vi "3D Omni Robot.vi"() -> ()   [LabVIEW 2015]
doc: "This example shows how to use the Steering VIs to define and simulate a dynamic model of a three-wheeled omnidirectional robot on a smooth surface."
uses:
  Robot Position.ctl
  <vilib>/robotics/Steering/Wheel/Wheel Parameters.ctl
  <vilib>/robotics/Steering/Wheel/Rotation Direction.ctl
  <vilib>/Simulation/Scripting/Companion Diagram/SimConfigNode/SimParams.ctl
  <vilib>/Simulation/Scripting/Companion Diagram/SimConfigNode/_simSolvers.ctl
  <vilib>/Simulation/Implementation/Shared/SIMSCR Execution Mode.ctl
  <vilib>/Platform/TimedLoop/XDataNode/timing_clust.ctl
  <vilib>/Platform/TimedLoop/XDataNode/nitl_modes.ctl
  <vilib>/Platform/TimedLoop/XDataNode/wakeup.ctl
  <vilib>/Simulation/Param Hierarchy/Typedefs/SIMPH Param Control Actions.ctl
  <vilib>/Simulation/Implementation/Shared/NILVSim_ParamChanged.vi
  <vilib>/Simulation/Implementation/Shared/NILVSim_FinishedLate.vi
  <vilib>/Simulation/Implementation/Shared/NILVSIM_BeginStep.vi
  <vilib>/Simulation/Utility/Implementation/SIM Halt.vi
  <vilib>/Simulation/Implementation/Shared/NILVSim_Manager.vi
  <vilib>/Utility/error.llb/Clear Errors.vi
  <vilib>/Simulation/Implementation/Shared/NILVSim_FinalizeModel.vi
  <vilib>/Analysis/coordinate.llb/2D Cartesian Coordinate Rotation.vi
  <vilib>/Analysis/coordinate.llb/2D Cartesian Coordinate Rotation (Scalar).vi
  <vilib>/robotics/Steering/Omnidirectional Wheel/Create Omnidirectional Wheel.vi
  <vilib>/robotics/Steering/Steering Frame/Create User Defined Steering Frame.vi
  <vilib>/Simulation/Implementation/Shared/SIM Unbundle Sim Info.vi
  <vilib>/Simulation/Implementation/Shared/SIMSH Read Queue.vi
  <vilib>/Simulation/Implementation/Shared/NILVSim_Initialize.vi
  <vilib>/Simulation/Utility/Implementation/NILVSim Get Time and IsAcceptedStep.vi
  <vilib>/Simulation/Implementation/Shared/NILVSim_GetModelError.vi
  <vilib>/Simulation/Implementation/Shared/SIM Bundle Sim Info.vi
  <vilib>/robotics/Steering/Steering Frame/Apply Steering Frame Velocity to Motors.vi
  <vilib>/robotics/Steering/Steering Frame/Get Steering Frame Velocity from Motors.vi
  <vilib>/Simulation/Scripting/Companion Diagram/SimConfigNode/SimDog.xnode
  Omni Robot Model.vi
  <vilib>/Platform/TimedLoop/XDataNode/XDataNode.xnode
  <vilib>/Simulation/Implementation/XNodeFramework/SimXNode/SimX.xnode
  <vilib>/robotics/Steering/Steering Frame/NI_Robotics_Steering Frame.lvclass
  <vilib>/robotics/Steering/Wheel/NI_Robotics_Wheel.lvclass
  <vilib>/robotics/Steering/Omnidirectional Wheel/NI_Robotics_Omnidirectional Wheel.lvclass
  <vilib>/Platform/TimedLoop/XDataNode/XDNodeRunTimeDep.lvlib
  <vilib>/Simulation/Implementation/Shared/NI_SIM_Implementation.lvlib
panel:
  in  "Velocity":T1(ring)
  out "motor states":dbl[](array[numeric]) format="%#.3f"
  in  "motor setpoints":dbl[](array[numeric])=[0.0, 0.0, 0.0] format="%#.3f"
  in  "reset":bool
  out "complete":bool
  in  "stop":bool
  out "robot position":T2 {"ccw wheel angles" format="%#.3f"; "global theta" format="%#.3f"; "global y" format="%#.3f"; "global x" format="%#.3f"}
  in  "Angular Velocity (rad/s)":dbl(slide) min=-1.0 max=1.0 scale=1.0..-1.0
  out "Angular Velocity Feedback":dbl(slide) scale=1.0..-1.0
  in  "Y Velocity (m/s)":dbl(slide) min=-1.0 max=1.0 scale=-1.0..1.0
  out "Y Velocity Feedback":dbl(slide) scale=-1.0..1.0
  in  "X Velocity (m/s)":dbl(slide) min=-1.0 max=1.0 scale=-1.0..1.0
  out "X Velocity Feedback":dbl(slide) scale=-1.0..1.0
  out "3D Picture":refnum<vi>(3d-picture)
  # "This VI simulates the steering of a three-wheeled omnidirectional robot on a smooth surface.\n\n1. Run the VI, then move the sliders to control the forward, lateral, and angular velocity components of the robot.\n\n2. Press the Reset Position button to move the robot back to its starting position."
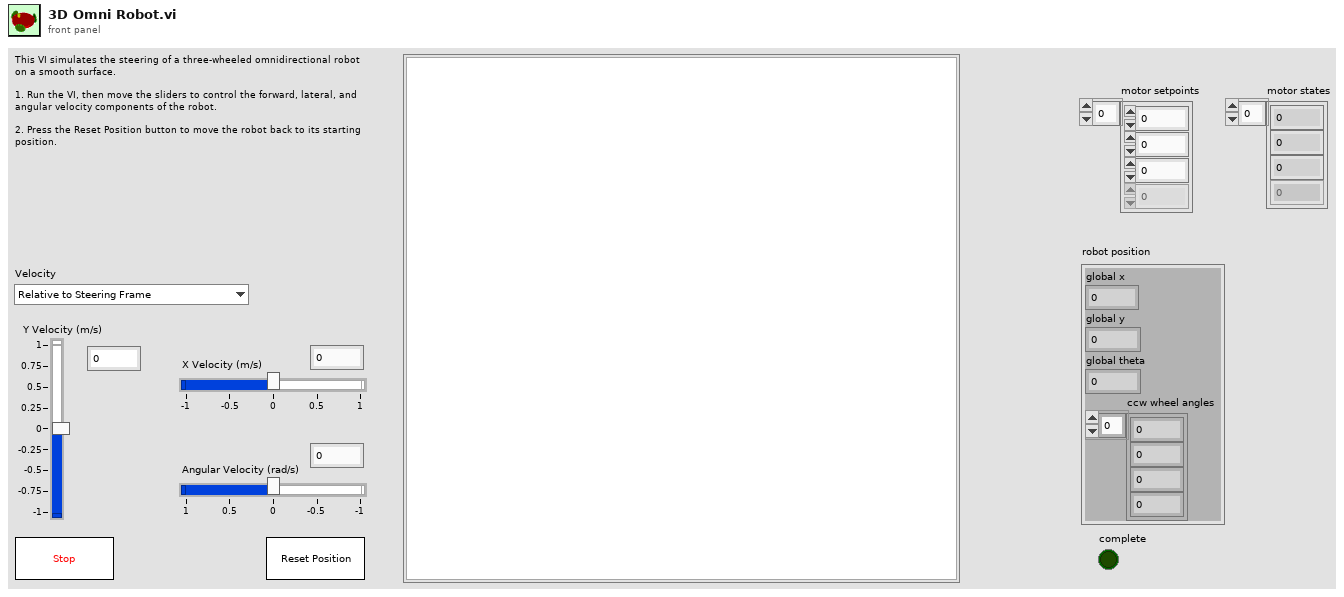
[diagram p1: front panel]
types:
  T1 = enum16{"Relative to Steering Frame", "Relative to Global Frame"}
  T2 = typedef "Robot Position.ctl" = cluster{"global x":dbl, "global y":dbl, "global theta":dbl, "ccw wheel angles":dbl[]}
  T3 = typedef "NI_Robotics_Wheel.lvclass/Rotation Direction.ctl" = u16
  T4 = typedef "NI_Robotics_Wheel.lvclass/Wheel Parameters.ctl" = cluster{"wheel radius":dbl, "gear ratio":dbl, "forward rotation direction":T3}
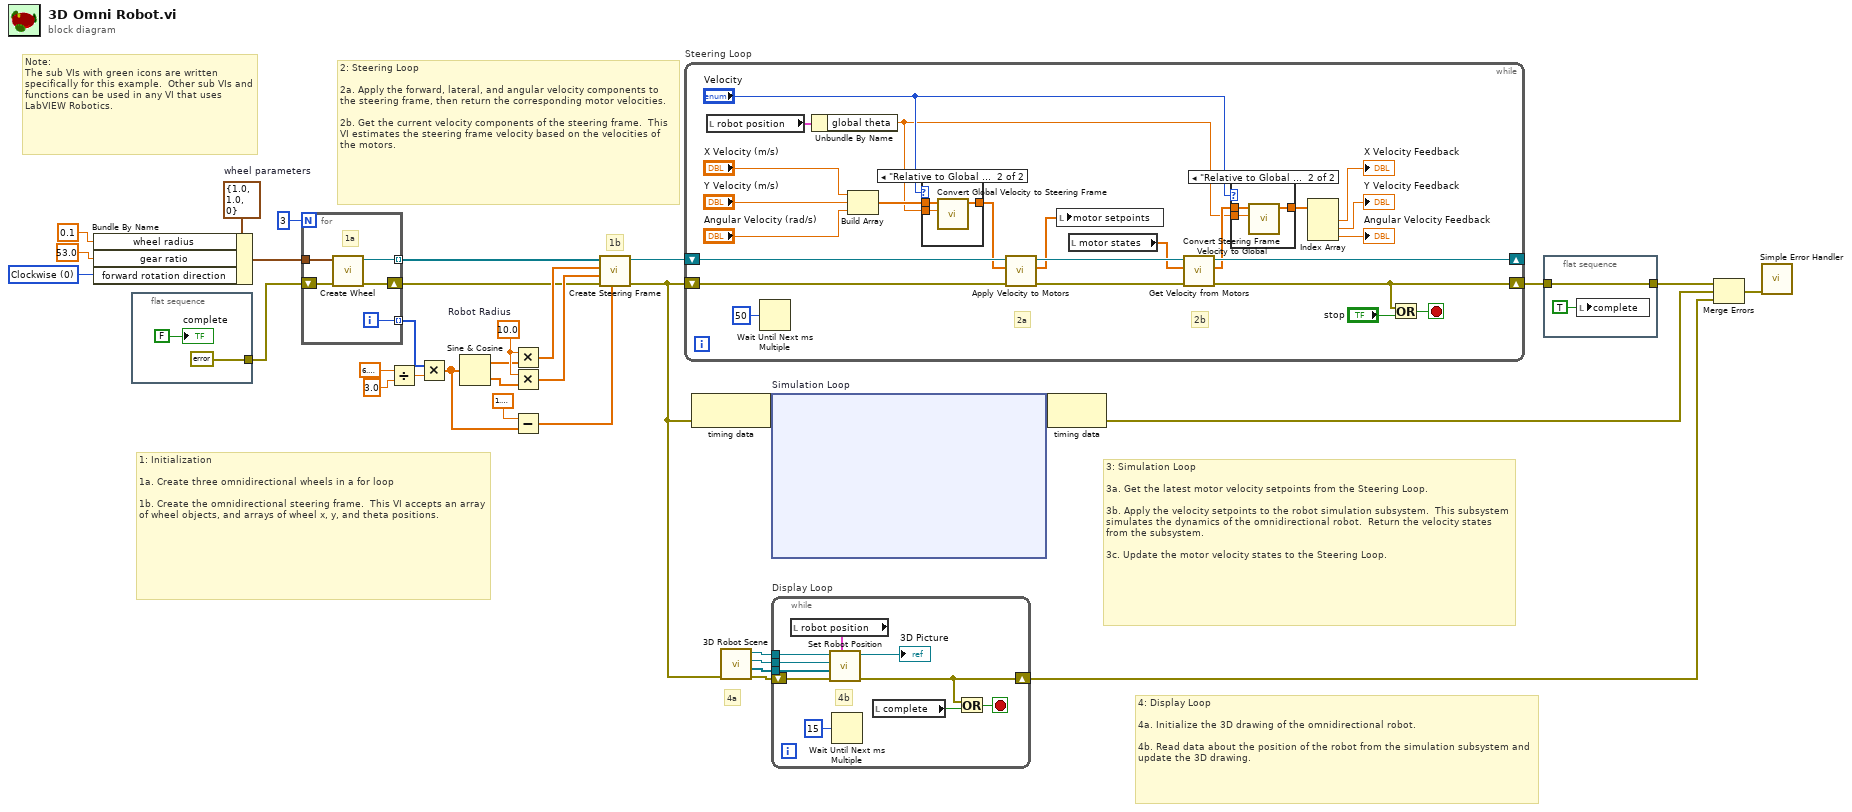
[diagram p0: block diagram]
diagram:
  w8 = T3 0 items=["Clockwise", "Counterclockwise"] ("forward rotation direction")
  w13 = 10.0  # Robot Radius
  w31 = T4 {"wheel radius"=1.0, "gear ratio"=1.0, "forward rotation direction"=0}  # wheel parameters
  # "3: Simulation Loop\n\n3a. Get the latest motor velocity setpoints from the Steering Loop.\n\n3b. Apply the velocity setpoints to the robot simulation subsystem.  This subsystem simulates the dynamics of the omnidirectional robot.  Return the velocity states from the subsystem.\n\n3c. Update the motor velocity states to the Steering Loop."
  # "Note:\nThe sub VIs with green icons are written specifically for this example.  Other sub VIs and functions can be used in any VI that uses LabVIEW Robotics."
  # "4a"
  # "4: Display Loop\n\n4a. Initialize the 3D drawing of the omnidirectional robot.\n\n4b. Read data about the position of the robot from the simulation subsystem and update the 3D drawing."
  # "2: Steering Loop\n\n2a. Apply the forward, lateral, and angular velocity components to the steering frame, then return the corresponding motor velocities.\n\n2b. Get the current velocity components of the steering frame.  This VI estimates the steering frame velocity based on the velocities of the motors."
  # "1b"
  # "1: Initialization\n\n1a. Create three omnidirectional wheels in a for loop\n\n1b. Create the omnidirectional steering frame.  This VI accepts an array of wheel objects, and arrays of wheel x, y, and theta positions."
  n1 = Bundle By Name(cluster=w31, "wheel radius"=0.1, "gear ratio"=53.0, "forward rotation direction"=w8) -> (w28:T4)
  n2 = flat-sequence {
    tunnel: [errorcluster {"status"=FALSE, "code"=0, "source"=""} ("error out")] -> w23
    frame #0 {
      "complete" <- FALSE ("complete")
    }
  }
  n3 = for {
    N: 3 -> [_]
    shift-right: [w40] -> w5
    shift-left: w23 -> [w41]
    tunnel: [w39] -> w18 mode=indexing
    tunnel: w28 -> [w38]
    tunnel: [w37] -> w14 mode=indexing
    i -> [w37]
    # "1a"
    n4 = call-poly <vilib>:"Create Wheel.vi"("error in (no error)"=w41, "wheel parameters"=w38) -> ("error out"=w40:errorcluster, "omni wheel out"=w39:refnum<class "NI_Robotics_Omnidirectional Wheel.lvclass">)  [unwired: 8 in]
  }
  n5 = Divide(x=6.283185307179586, y=3.0) -> (x/y=w15:dbl)
  n6 = Multiply(x=w14, y=w15) -> (x*y=w3:dbl[])
  n7 = Sine & Cosine(0:w3) -> (1:w2:dbl[], 2:w1:dbl[])
  n8 = Multiply(x=w13, y=w2) -> (x*y=w12:dbl[])
  n9 = Multiply(x=w13, y=w1) -> (x*y=w11:dbl[])
  n10 = Subtract(x=1.5707963267948966, y=w3) -> (x-y=w9:dbl[])
  n11 = call-poly <vilib>:"Create Steering Frame.vi"("wheel frame angles (rad)"=w9, "error in (no error)"=w5, "wheel y positions"=w11, "wheel x positions"=w12, "wheels"=w18) -> ("error out"=w4:errorcluster, "steering frame out"=w32:refnum<class "NI_Robotics_Steering Frame.lvclass">)  [unwired: 5 in]
  n12 = while "Steering Loop" {
    shift-right: [w52] -> _
    shift-left: w32 -> [w55]
    shift-right: [w42] -> w24
    shift-left: w4 -> [w54]
    stop <- w57 stop-if-true
    # "2b"
    # "2a"
    n13 = local read "robot position"() -> (w44:T2)
    n14 = Wait Until Next ms Multiple(millisecond multiple=u32 50) -> ()  [unwired: 1 out]
    n15 = Unbundle By Name(w44) -> ("global theta"=w43:dbl)
    n16 = Build Array("X Velocity (m/s)", "Y Velocity (m/s)", "Angular Velocity (rad/s)") -> (w48:dbl[])
    n17 = case shown="\"Relative to Global Frame\"" "Velocity" {
      tunnel: w48 -> [w70 w73]
      tunnel: [w70 w72] -> w47
      tunnel: w43 -> [_ w71]
      frame "Relative to Steering Frame", Default {
      }
      frame "Relative to Global Frame" {
        n18 = call <vilib>:"Convert Global Velocity to Steering Frame.vi"("steering frame angle (rad)"=w71, "global velocity"=w73) -> ("steering frame velocity"=w72:dbl[])  [unwired: 9 in]
      }
    }
    n19 = call-poly <vilib>:"Apply Velocity to Motors.vi"("error in (no error)"=w54, "steering frame velocity"=w47, "steering frame in"=w55) -> ("error out"=w53:errorcluster, "ccw motor velocity setpoints"=w51:dbl[], "steering frame out"=w56:refnum<class "NI_Robotics_Steering Frame.lvclass">)  [unwired: 4 in, 2 out]
    n20 = local write "motor setpoints"(w51) -> ()
    n21 = local read "motor states"() -> (w50:dbl[])
    n22 = call-poly <vilib>:"Get Velocity from Motors.vi"("error in (no error)"=w53, "ccw motor velocity states"=w50, "steering frame in"=w56) -> ("error out"=w42:errorcluster, "estimated steering frame velocity"=w46:dbl[], "steering frame out"=w52:refnum<class "NI_Robotics_Steering Frame.lvclass">)  [unwired: 6 in]
    n23 = case shown="\"Relative to Global Frame\"" "Velocity" {
      tunnel: w46 -> [w66 w69]
      tunnel: [w66 w68] -> w45
      tunnel: w43 -> [_ w67]
      frame "Relative to Steering Frame", Default {
      }
      frame "Relative to Global Frame" {
        n24 = call <vilib>:"Convert Steering Frame Velocity to Global.vi"("steering frame angle (rad)"=w67, "steering frame velocity"=w69) -> ("global velocity"=w68:dbl[])  [unwired: 9 in]
      }
    }
    n25 = Index Array(array=w45) -> (element #1=→"X Velocity Feedback":dbl, element #2=→"Y Velocity Feedback":dbl, element #3=→"Angular Velocity Feedback":dbl)  [unwired: 3 in]
    n26 = Or(x=w42, y="stop") -> (x .or. y?=w57:bool)
  }
  n27 = node-c288(w4) -> (w34:variant)
  n28 = call "3D Robot Scene.vi"("error in (no error)"=w4) -> ("error out"=w20:errorcluster, "axles"=w25:refnum<vi>[], "robot"=w26:refnum<vi>, "scene"=w27:refnum<vi>)  [unwired: 7 in]
  n29 = node-c254 "Simulation Loop"(w34) -> (w33:variant)
  n30 = while "Display Loop" {
    tunnel: w27 -> [w77]
    tunnel: w26 -> [w78]
    tunnel: w25 -> [w79]
    shift-right: [w74] -> w19
    shift-left: w20 -> [w80]
    stop <- w75 stop-if-true
    # "4b"
    n31 = local read "robot position"() -> (w81:T2)
    n32 = call "Set Robot Position.vi"("robot position"=w81, "error in (no error)"=w80, "axles"=w79, "robot"=w78, "scene"=w77) -> ("error out"=w74:errorcluster, "scene out"=→"3D Picture":refnum<vi>)  [unwired: 5 in]
    n33 = Wait Until Next ms Multiple(millisecond multiple=u32 15) -> ()  [unwired: 1 out]
    n34 = local read "complete"() -> (w76:bool)
    n35 = Or(x=w74, y=w76) -> (x .or. y?=w75:bool)
  }
  n36 = node-c288(w33) -> (w6:errorcluster)
  n37 = flat-sequence {
    tunnel: w24 -> [w84]
    tunnel: [w84] -> w22
    frame #0 {
      n38 = local write "complete"(TRUE ("complete")) -> ()
    }
  }
  n39 = Merge Errors(w22, w6, w19) -> (w21:errorcluster)
  n40 = call <vilib>:"Simple Error Handler.vi"("error in (no error)"=w21) -> ()  [unwired: 4 in, 5 out]
